vi "AlliGator Phasor ROI to Source Image ROI.vi"(8 "Error In":errorcluster, 10 "Phasor Plot ROI":T2, 11 "AlliGator IV DVR in":refnum<data-value>) -> (0 "Error Out":errorcluster, 1 "Message":string, 2 "Source Image ROI":T1 {"Contours"."Type" items=["No Selection", "Point", "Line", "Rectangle", "Oval", "Polygon", "Freehand Region", "Annulus", "Unused2", "Unused3", "Broken Line", "Freehand Line", "Rotated Rectangle"]}, 3 "AlliGator IV DVR out":refnum<data-value>, 4 "CPU (s)":dbl)   [LabVIEW 2021, in "AlliGator Phasor Plot.lvlib"]
doc: "Buils a Source Image ROI comprising all pixels whose phasors are included in the Phasor Plot ROI."
uses:
  AlliGator Phasor Plot.lvlib
  Internal Variables/AlliGator Internal Variables v2.ctl
  <vilib>/vision/Image Controls.llb/IMAQ Image.ctl
  Internal Variables/AlliGator Gate Image Set.ctl
  Files/AlliGator FLI Dataset Type.ctl
  Files/AlliGator Data Series Type.ctl
  Dual-Channel Datasets/AlliGator Dataset Channel.ctl
  Settings/AlliGator Gate Arithmetic.ctl
  Source Image/AlliGator Displayed Image.ctl
  Image/Named ROI Description.ctl
  Phasor Graph/AlliGator Decay Metadata v3.ctl
  Decay Analysis/Decay Preprocessing/AlliGator Decay Background Subtraction Info.ctl
  Decay Analysis/Decay Preprocessing/AlliGator Baseline Subtraction Method.ctl
  Graphs/XY Graph/XY Graph Plot Shift Parameters.ctl
  Graphs/XY Graph/XY Graph Plot Shift Method.ctl
  Decay Analysis/Decay Preprocessing/AlliGator Decay Extrapolation Parameters.ctl
  Phasor/Calibration Phasor (m, phi).ctl
  Phasor/Phasor Reference Series.ctl
  Phasor/Phasor Calibration Map v2.ctl
  Phasor/Phasor (g, s).ctl
  Phasor Graph/AlliGator Raw Phasor Plot Data v4.ctl
  Phasor/Phasor Standard Deviation Options.ctl
  AlliGator Phasor Multi-Harmonic Data.ctl
  Phasor/Phasor Harmonic Data.ctl
  Decay Fit Parameter Map/AlliGator Decay Fit Options & Parameters v2.ctl
  Fits/IRF(X)PSED/Decay Fit Options v2.ctl
  Fits/Decay Convolution/Decay Model.ctl
  Fits/Residual Type.ctl
  Fits/IRF(X)PSED/Fit Weights Type.ctl
  Fits/Non-linear Fitting Method v2.ctl
  Fits/Fit Calculation Method.ctl
  Fits/Non-linear Fitting Algorithm.ctl
  Decay Analysis/Decay Fit/AlliGator Decay Fit Parameter Constraints 2.ctl
  Fits/IRF(X)PSED/Decay Fit Parameters In List.ctl
  Fits/IRF(X)PSED/MLE Baseline Offset Type.ctl
  Decay Analysis/Decay Preprocessing/AlliGator Decay Preprocessing Parameters.ctl
  Fits/IRF(X)PSED/Decay Fit Parameters & Derived Quantities List v2.ctl
  Decay Fit Parameter Map/AlliGator Parameter Maps Data.ctl
  Globals, Variables, Constants/AlliGator Variables List.ctl
  Phasor Ratio/AlliGator Phasor Plot Reference Points.ctl
  9cfa6bdc-d1e0-4e6c-94b8-050a3d16fc11.vi
  <vilib>/vision/NI_Vision_Development_Module.lvlib
  Globals, Variables, Constants/AlliGator Globals, Variables & Constants.lvlib
  Phasor Ratio/AlliGator Phasor Ratio.lvlib
  Time/Time.lvlib
  Utilities/Utilities.lvlib
  Image/Image.lvlib
  Phasor/Phasor.lvlib
  Decay Analysis/Decay Preprocessing/AlliGator Decay Preprocessing.lvlib
  Graphs/XY Graph/XY Graph Add-Ons.lvlib
  Phasor Graph/AlliGator Phasor Graph.lvlib
  Files/AlliGator Files.lvlib
  Source Image/AlliGator Source Image.lvlib
  Internal Variables/AlliGator Internal Variables.lvlib
  Fits/Fits.lvlib
  Decay Analysis/Decay Fit/AlliGator Decay Fit.lvlib
  Decay Fit Parameter Map/AlliGator Decay Fit Parameter Map.lvlib
  Settings/AlliGator Settings.lvlib
  Dual-Channel Datasets/AlliGator Dual-Channel Datasets.lvlib
panel:
  # "see the AlliGator License on the block diagram (Ctrl+E or Window:Show Block Diagram)"
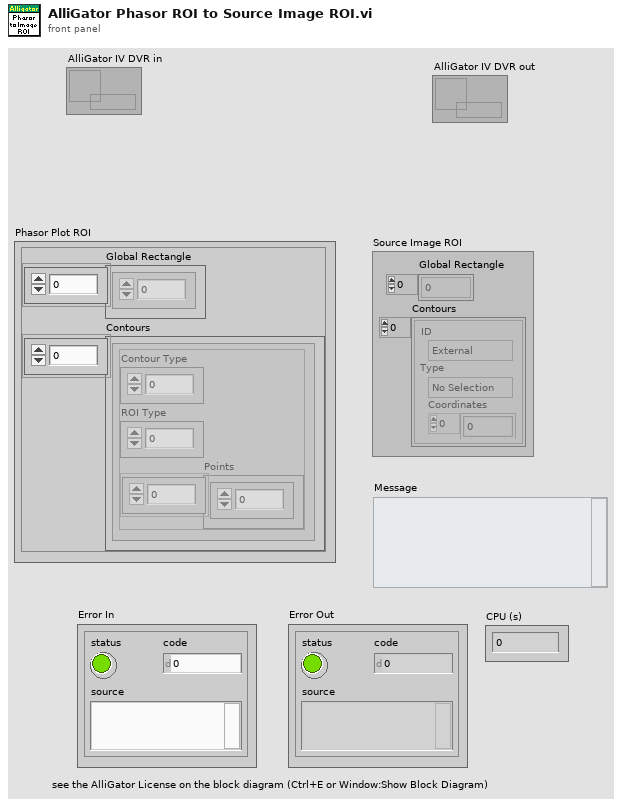
[diagram p1: front panel]
types:
  T1 = typedef "ROI Descriptor" = cluster{"Global Rectangle":i32[], "Contours":cluster{"ID":enum32{"External", "Internal"}, "Type":u32, "Coordinates":i32[]}[]}
  T2 = cluster{"Global Rectangle":i32[], "Contours":cluster{"Contour Type":u32, "ROI Type":u32, "Points":i32[]}[]}
  T3 = typedef "AlliGator Phasor Ratio.lvlib/AlliGator Phasor Plot Reference Points.ctl" = cluster{"O_h":dbl, "O_v":dbl, "1_h":dbl, "1_v":dbl}
  T4 = typedef "AlliGator Globals, Variables & Constants.lvlib/AlliGator Variables List.ctl" = enum16{"---- GUI ----", "GUI:Initialization Status", "GUI:State Indicators Refnum", "GUI:Original AlliGator Menu Items", "GUI:Current Action Loop State", "GUI:Script in progress", "GUI:Playback", "GUI:Loop Playback", "GUI:Search ROI Used", "GUI:Search ROI", "Decay Graph Max Legend Size", "Intensity Graph Max Legend Size", "Decay Statistics Graph Max Legend Size", "Phasor Graph Max Legend Size", "Phasor Ratio Graph Max Legend Size", "Lifetime Graph Max Legend Size", "---- Files ----", "Files:Export Dataset Frames as Individual Files", "Files:Show Batch Export Help Balloons", "Files:Frames in Dataset", "Files:ptu File Frame Start Indices", "Files:Current Frame in Dataset", "Files:Current Frame Timestamp", "Files:Dataset Loaded", "Files:Dataset Metadata", "Files:Dataset Channel", "Files:Dataset Data Description", "Files:Background Dataset Metadata", "Files:Background Dataset Channel", "Files:Background Dataset Data Description", "Files:Background File Subtraction", "Files:Background File Path", "Files:Background File Pile-up Correction", "Files:Background File Pixel Well Capacity", "Files:Background File Scaling Factor", "Files:Current Dataset Load Settings", "Files:Dataset Path", "Files:ICCD-specific Information", "Files:Macrotime Gate Separation", "------ Python Plugins ------", "Python Plugins:Information", "Python Plugins:Python Session", "Python Plugins:Valid Python Session?", "---- Source Image ----", "Source Image:ROIs", "Source Image:Current ROI", "Source Image:ROI Event Refnum", "X_Source Image Display Range", "X_Source Image Palette Information", "X_Type of Displayed Image", "X_Time Gate Slider", "Source Image:Palette List", "Source Image:Scale", "Source Image:ROI Overlay Color", "Source Image:Overlay to Erase", "Source Image:Is Displayed Image Accumulated", "Source Image:White Light Image Modified", "Source Image:Mask Image Modified", "---- Image Profile Window ----", "Image Profile:Window Event Refnum", "Image Profile:IntensityType", "Image Profile:Intensity Average Type", "Image Profile:Intensity-weighted SDV", "Image Profile:Box Profile Type", "Image Profile:Window Open", "Image Profile:Plotted Fit Parameter", "------ Phasor Graph -------", "Phasor Graph:Show Line", "---- Phasor Plot ---", "Phasor Plot:Parameters Changed", "Phasor Plot:FLI Dataset Modified since last Calculation", "Phasor Harmonics Data", "Selected Phasor Harmonics", "Phasor Harmonic Manager Event Refnum", "Phasor Plot:ROIs", "Phasor Plot:Current ROI", "Phasor Plot:ROI Event Refnum", "Phasor Plot:Image Reference Points", "Phasor Plot:Computed", "Phasor Plot:Palette Information", "Phasor Plot:Palette List", "Phasor Plot:Phasor Ratio Palette Information", "Phasor Plot:Phasor Ratio Palette List", "Phasor Plot:Image Scale", "Phasor Plot:Image Overlay to Erase", "Phasor Plot:Image Elements to Update", "Phasor Plot:Current Calculation Parameters", "Phasor Plot:Current Calibration Options", "Phasor Plot:Reset Cumulated Phasor Plot", "Phasor Plot:Reference 1", "Phasor Plot:Lifetime Reference 1", "Phasor Plot:Reference 1 Frequency", "Phasor Plot:Reference 2", "Phasor Plot:Lifetime Reference 2", "Phasor Plot:Reference 2 Frequency", "---- Decay Analysis ----", "Number of Selected Decays to Fit", "LS Fit Results", "LAR Fit Results", "BS Fit Results", "Last Decay Max - Min", "Best Fit Parameters", "Best Fit Parameter Names", "Actual Size X", "Actual Size Y", "Binning X", "Binning Y", "Actual # Gates", "Dataset Number", "Gates to...", "Gates Skipped", "Gates to keep", "Gate Step", "Gate Separation", "Reversed Gates", "Pile-up Correction", "Pixel Well Capacity", "Background Subtracted", "Background Subtraction Method", "Background Definition Range", "Background File (deprecated)", "Number of Dataset Accumulated", "Array of Accumulated Dataset Paths", "Do Averaged Datasets", "Destination File Path", "Process Plot Target", "Use 1/D as Phasor Frequency", "---- Decay Fit Parameter Map -----", "Decay Fit Parameter Map:Palette Information", "Decay Fit Parameter Map:Palette List", "---- Parameter Map ----", "Parameter Map:Palette Information", "Parameter Map:Palette List", "------- Local Decay Window ---------", "Local Decay Graph Window:Event Refnum", "Local Decay Graph Window:Use normalized IRF for convolution", "----- Miscellaneous ----", "Misc:Skippable Dialog Windows Status"}
  T5 = typedef "AlliGator Internal Variables.lvlib/AlliGator Internal Variables v2.ctl" = cluster{"Displayed Image":T6, "White Light Image":T6, "Mask Image":T6, "ROI Mask Image":T6, "Current Dataset Images 1":T7, "Background Dataset Images 1":T7, "Current Dataset Images 2":T7, "Background Dataset Images 2":T7, "Current Dataset Arithmetic Images":T7, "Accumulated Dataset Images 1":T7, "Accumulated Dataset Images 2":T7, "Accumulated Dataset Arithmetic Images":T7, "Phasor Plot Image":T6, "Decay Fit Parameter Map Image":T6, "Parameter Map Image":T6, "Single Data Point Path":path, "White Light Image Path":path, "Mask Image Path":path, "Time-Series Folder":path, "[Time-Series Paths]":path[], "Current Dataset":i32, "Single Dataset Type":T8, "Current Folder":string, "AlliGator Data Series Type":T9, "# Datasets":i32, "Dual-Channel Dataset":bool, "Selected Channel Name":string, "Dataset Channel":T10, "Channel Arithmetic":T11, "Dual-Channel Background Dataset":bool, "Background Channel":T10, "Dual-Channel Accumulated Dataset":bool, "Start Time":dbl, "[Time-Series Timestamps]":dbl[], "[Intensity Corrections]":dbl[], "Time Series Script":bool, "Type of Displayed Image":T12, "Gate Image Slide":u16, "# Gates":i32, "ROIs":T13[], "ROI Decay":cluster{"t Array":dbl[], "I Array":dbl[]}, "Valid Decay":bool, "Decay  Metadata":T14, "Reference Decay Plot Name":string, "Reference Decay":cluster{"t Array":dbl[], "I Array":dbl[]}, "Decay Shift Plot":cluster{"Time Stamps":dbl[], "Decay Shifts":dbl[]}, "[Decays Max Values]":sgl[], "[Decays Min Values]":sgl[], "Calibration Phasor":T20, "Calibration Phasor Series":T21, "Phasor Calibration Map":T22, "Calibration Map MD5 Digest":string, "Last Raw Phasor":T23, "Last Calibrated Phasor":T23, "Last Calibrated Phasor SDV":T23, "Phasor Graph:Phasor Plot":cluster{"g Array":dbl[], "s Array":dbl[]}, "Phasor Graph:Phasor SDV Plot":cluster{"g Array":dbl[], "s Array":dbl[]}, "[Phasor Graph:Raw Phasor Plots]":T24[], "Phasor Plot locked to Ref 1":i32, "[Phasor Plot(s) locked to Ref 1]":i32[], "[Phasor Plot(s) locked to Ref 2]":i32[], "[Pixel Phasors]":T23[], "[[Sum Image]]":dbl[][], "[[CSG Phasors]]":csg[][], "[[Valid Pixel?]]":bool[][], "I/m/phi Dataset":cluster{"I/m/phi Dataset?":bool, "Base Frequency":dbl[unit], "Harmonic Orders":u8[]}, "Multi Phasor Plot Data":T26, "Decay Fit Options & Parameters":T28, "Fit Options: Decay Preprocessing Parameters":T39, "Fit Options: Reference Decay":cluster{"t Array":dbl[], "I Array":dbl[]}, "Is Full Image Parameters Map":bool, "Is Single-Pixels Parameters Map":bool, "NLSF Parameters Map X Resolution":i32, "NLSF Parameters Map Y Resolution":i32, "[Single Decay Fit Parameters]":dbl[], "Fit Model":T30, "[[Multiple Decays Fit Parameters]]":dbl[][], "[[Multiple Decays Fit Parameter SDVs]]":dbl[][], "[[IRFs]]":dbl[][], "IRF Array Time Axis":dbl[], "Decay Array Time Axis":dbl[], "[Decay Fit Parameter Names]":T40[], "[[Phasor Ratios]]":dbl[][], "[[Average Lifetimes]]":dbl[][], "Amplitude Weighted Average Lifetime":bool, "[Decay Sum]":dbl[], "[Map Set Names]":string[], "[Parameter Maps]":T41[], "[[User-defined Quantities]]":dbl[][], "User-defined Quantity":string}
  T6 = typedef "IMAQ Image.ctl" = refnum<image>
  T7 = typedef "AlliGator Internal Variables.lvlib/AlliGator Gate Image Set.ctl" = cluster{"SGL Image Max":T6, "SGL Image Sum":T6, "SGL Gate Images":T6[], "SGL Image Min":T6}
  T8 = typedef "AlliGator Files.lvlib/AlliGator FLI Dataset Type.ctl" = enum16{"HDF5 FLI Dataset", "Gate Image Folder", ".sdt FLI Dataset (Becker & Hickl)", ".ptu FLI Dataset (PicoQuant)", "SS1 FLI Dataset", "SS2 FLI Dataset", "I/m/phi Dataset", ".bin FLI Dataset (PicoQuant Binned)", ".bin FLI Dataset (Piccolo Binned)"}
  T9 = typedef "AlliGator Files.lvlib/AlliGator Data Series Type.ctl" = enum16{"Not a Supported Series", "Gate Images Folder Series", "SwissSPAD 2 Dataset Series", "B&H FLI Dataset Series", "PicoQuant PTU FLI Dataset Series", "PicoQuant BIN FLI Dataset Series", "Piccolo hist BIN FLI Dataset Series", "HDF5 FLI Dataset Series"}
  T10 = typedef "AlliGator Dual-Channel Datasets.lvlib/AlliGator Dataset Channel.ctl" = enum16{"G2", "INT"}
  T11 = typedef "AlliGator Settings.lvlib/AlliGator Gate Arithmetic.ctl" = enum16{"None", "INT-G2", "G2/INT*<INT>", "(1 - G2/INT)*<INT>"}
  T12 = typedef "AlliGator Source Image.lvlib/AlliGator Displayed Image.ctl" = enum16{"Single Gate", "Sum of All Gates", "Max of All Gates", "Min of All Gates", "-", "White Ligth Image", "Mask Image"}
  T13 = typedef "Image.lvlib/Named ROI Description.ctl" = cluster{"ROI Descriptor":T1, "ROI Name":string, "Overlay Color":u32}
  T14 = typedef "AlliGator Phasor Graph.lvlib/AlliGator Decay Metadata v3.ctl" = cluster{"ROI Descriptor":T1, "ROI Center":cluster{"X":i32, "Y":i32}, "Decay Background Subtraction Info":T15, "Decay Reverted":bool, "Decay Smoothened":bool, "Decay Straightened":bool, "Fitted Tau (Decay Straightening)":dbl, "Decay Shift Parameters":T17, "Decay Shifted":bool, "Decay Extrapolated":bool, "Decay Extrapolation Parameters":T19, "Decay Normalized":bool, "Fold Decay":bool, "# Folds":u32}
  T15 = typedef "AlliGator Decay Preprocessing.lvlib/AlliGator Decay Background Subtraction Info.ctl" = cluster{"Laser Period":dbl[unit], "Gate Duration":dbl[unit], "Baseline Subtraction Method":T16, "Background Definition Range":cluster{"Min Gate":dbl[unit], "Max Gate":dbl[unit]}, "Total Intensity w/o Bkgd Subtraction":dbl, "Bkgd-subtracted Intensity (exp)":dbl, "# Data Points":i32, "Background/Gate":dbl, "Fitted Lifetime":dbl[unit], "Bkgd-subtracted Intensity (theo)":dbl}
  T16 = typedef "AlliGator Decay Preprocessing.lvlib/AlliGator Baseline Subtraction Method.ctl" = enum16{"Mean", "Min", "Square Gated Single-Exponential", "File", "Constant"}
  T17 = typedef "XY Graph Add-Ons.lvlib/XY Graph Plot Shift Parameters.ctl" = cluster{"Type":T18, "Shift":dbl[unit], "Threshold":dbl, "Rotate":bool}
  T18 = typedef "XY Graph Add-Ons.lvlib/XY Graph Plot Shift Method.ctl" = enum16{"Default", "CFD", "Threshold", "Cross-Correlation"}
  T19 = typedef "AlliGator Decay Preprocessing.lvlib/AlliGator Decay Extrapolation Parameters.ctl" = cluster{"Additional Points":u32, "Head Fraction":dbl, "Fitted Tau":dbl, "Use Periodicity":bool, "Use Cursors":bool, "Tail Fraction":dbl}
  T20 = typedef "Phasor.lvlib/Calibration Phasor (m, phi).ctl" = cluster{"m":dbl, "phi":dbl, "Phasor Frequency":dbl[unit], "Reference Lifetime":dbl[unit]}
  T21 = typedef "Phasor.lvlib/Phasor Reference Series.ctl" = cluster{"m Array":dbl[], "phi Array":dbl[], "Phasor Frequency":dbl[unit], "Calibration Lifetime":dbl[unit]}
  T22 = typedef "Phasor.lvlib/Phasor Calibration Map v2.ctl" = cluster{"Phasor Frequency":dbl[unit], "Calibration Lifetime":dbl[unit], "ROI Centers":cluster{"X":i32, "Y":i32}[], "ROI Descriptors":T1[], "Map Resolution X":i32, "Map Resolution Y":i32, "z Array":cdb[]}
  T23 = typedef "Phasor.lvlib/Phasor (g, s).ctl" = cluster{"g":dbl, "s":dbl}
  T24 = typedef "AlliGator Phasor Graph.lvlib/AlliGator Raw Phasor Plot Data v4.ctl" = cluster{"Phasor Plot Name":string, "Raw Phasor Plot":T23[], "Phasor Frequency":dbl[unit], "[Decay Metadata]":T14[], "Raw Phasor Plot SDV":T23[], "Phasor SDV Options":T25, "[Calibration Phasor]":T20[]}
  T25 = typedef "Phasor.lvlib/Phasor Standard Deviation Options.ctl" = cluster{"Compute Estimated SDV":bool, "# Replicas":u32, "Use Estimated Average Phasor":bool}
  T26 = typedef "AlliGator Phasor Plot.lvlib/AlliGator Phasor Multi-Harmonic Data.ctl" = cluster{"Base Frequency":dbl[unit], "# Harmonics":u8, "Harmonic Orders":u8[], "Phasor Plot Settings Checksum":u64, "Phasor Harmonic Data Array":T27[]}
  T27 = typedef "Phasor.lvlib/Phasor Harmonic Data.ctl" = cluster{"Phasor Harmonic Name":string, "Phasor Plot Settings Checksum":u64, "Phasor Frequency":dbl[unit], "Base Frequency":dbl[unit], "Harmonic Order":u8, "Phasor Plot Parameters":string, "Phasor Array [[CSG]]":csg[][], "Dataset File Path":path}
  T28 = typedef "AlliGator Decay Fit Parameter Map.lvlib/AlliGator Decay Fit Options & Parameters v2.ctl" = cluster{"SYNC Period":dbl[unit], "Fit Options":T29, "Fit Parameter Constraints":T36[], "MLE Baseline Offset":dbl, "MLE Baseline Offset Type":T38}
  T29 = typedef "Fits.lvlib/Decay Fit Options v2.ctl" = cluster{"Show Fit Residuals":bool, "Fit Model":T30, "Residual Type":T31, "Max Decay Percentile":dbl, "Min Decay Percentile":dbl, "Show Full Decay":bool, "Weights":T32, "Fitting Method":T33, "Compute Parameter Uncertainties":bool, "Periodic Boundaries":bool, "Model Calculation":T34, "Period":dbl[unit], "Termination Criteria":cluster{"Max Iterations":i32, "Max Function Calls":i32, "Max Time":dbl[unit], "Function Tolerance":dbl, "Parameter Tolerance":dbl, "Gradient Tolerance":dbl, "Min Lambda":dbl, "Max Lambda":dbl, "Initial Tick Count":u32}, "Offset Resolution":dbl[unit], "Use Local IRF":bool, "Fitting Algorithm":T35}
  T30 = typedef "Fits.lvlib/Decay Model.ctl" = enum16{"1-Exponential", "2-Exponentials"}
  T31 = typedef "Fits.lvlib/Residual Type.ctl" = enum16{"Standard", "Normalized", "Reduced"}
  T32 = typedef "Fits.lvlib/Fit Weights Type.ctl" = enum16{"Unweighted", "1/Variance", "Best of All"}
  T33 = typedef "Fits.lvlib/Non-linear Fitting Method v2.ctl" = enum16{"Least Square", "Least Absolute Residual", "Bisquare", "MLE", "-", "Best of All"}
  T34 = typedef "Fits.lvlib/Fit Calculation Method.ctl" = enum16{"Simulation", "Convolution", "Integration"}
  T35 = typedef "Fits.lvlib/Non-linear Fitting Algorithm.ctl" = enum16{"Levenberg-Marquardt", "Trust-Region Dogleg"}
  T36 = typedef "AlliGator Decay Fit.lvlib/AlliGator Decay Fit Parameter Constraints 2.ctl" = cluster{"Fit Parameter":T37, "Min Value":dbl, "Max Value":dbl, "Global":bool, "Used":bool}
  T37 = typedef "Fits.lvlib/Decay Fit Parameters In List.ctl" = enum16{"Offset", "Baseline", "A_1", "tau_1", "A_2", "tau_2"}
  T38 = typedef "Fits.lvlib/MLE Baseline Offset Type.ctl" = enum32{"Absolute", "Percentage"}
  T39 = typedef "AlliGator Decay Preprocessing.lvlib/AlliGator Decay Preprocessing Parameters.ctl" = cluster{"Background Subtraction":bool, "Straighten Decay":bool, "Reverse Gates":bool, "1-Normalized Decay":bool, "Smoothen Decay":bool, "Smoothing Parameter":dbl, "Shift Decay":bool, "Decay Shift Parameters":T17, "Extrapolate Decay":bool, "Additional Points":u32, "Head Fraction":dbl, "Pixel-Normalize Decay":bool, "Use Periodicity":bool, "Use Cursors":bool, "Tail Fraction":dbl, "Use Decay Pre-Processing":bool, "Fold Decay":bool, "# Folds":u32, "[0-1]-Normalized Decay":bool}
  T40 = typedef "Fits.lvlib/Decay Fit Parameters & Derived Quantities List v2.ctl" = enum16{"Offset", "Baseline", "A_1", "tau_1", "A_2", "tau_2", "<tau>_a", "f1_a", "f2_a", "<tau>_i", "f1_i", "f2_i", "-", "R^2", "Chi^2"}
  T41 = typedef "AlliGator Decay Fit Parameter Map.lvlib/AlliGator Parameter Maps Data.ctl" = cluster{"Map Set Name":string, "[Parameter Names]":string[], "[[Parameters]]":dbl[][], "[[Parameter SDVs]]":dbl[][], "Decay Array Time Axis":dbl[], "[[IRFs]]":dbl[][], "IRF Array Time Axis":dbl[]}
  T42 = typedef "Image Type" = u32
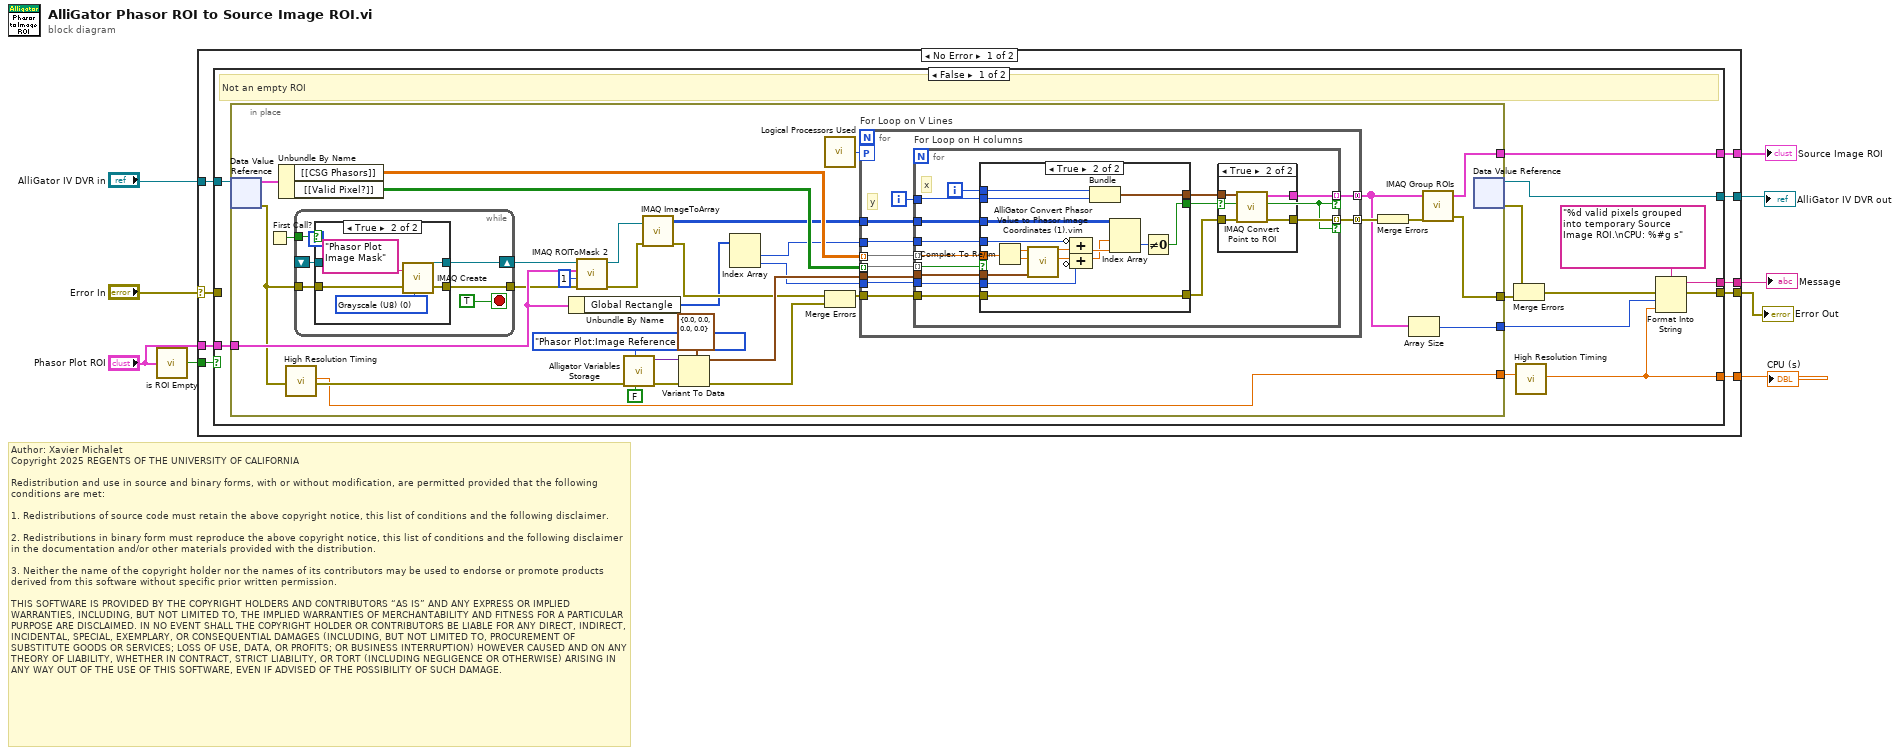
[diagram p0: block diagram]
diagram:
  # "Author: Xavier Michalet\nCopyright 2025 REGENTS OF THE UNIVERSITY OF CALIFORNIA\n\nRedistribution and use in source and binary forms, with or without modification, are permitted provided that the following conditions are met:\n\n1. Redistributions of source code must retain the above copyright notice, this list of conditions and the following disclaimer.\n\n2. Redistributions in binary form must reproduce the above copyright notice, this list of conditions and the following disclaimer in the documentation and/or other materials provided with the distribution.\n\n3. Neither the name of the copyright holder nor the names of its contributors may be used to endorse or promote products derived from this software without specific prior written permission.\n\nTHIS SOFTWARE IS PROVIDED BY THE COPYRIGHT HOLDERS AND CONTRIBUTORS “AS IS” AND ANY EXPRESS OR IMPLIED WARRANTIES, INCLUDING, BUT NOT LIMITED TO, THE IMPLIED WARRANTIES OF MERCHANTABILITY AND FITNESS FOR A PARTICULAR PURPOSE ARE DISCLAIMED. IN NO EVENT SHALL THE COPYRIGHT HOLDER OR CONTRIBUTORS BE LIABLE FOR ANY DIRECT, INDIRECT, INCIDENTAL, SPECIAL, EXEMPLARY, OR CONSEQUENTIAL DAMAGES (INCLUDING, BUT NOT LIMITED TO, PROCUREMENT OF SUBSTITUTE GOODS OR SERVICES; LOSS OF USE, DATA, OR PROFITS; OR BUSINESS INTERRUPTION) HOWEVER CAUSED AND ON ANY THEORY OF LIABILITY, WHETHER IN CONTRACT, STRICT LIABILITY, OR TORT (INCLUDING NEGLIGENCE OR OTHERWISE) ARISING IN ANY WAY OUT OF THE USE OF THIS SOFTWARE, EVEN IF ADVISED OF THE POSSIBILITY OF SUCH DAMAGE."
  n1 = call "is ROI Empty.vi"("Current ROI Descriptor"="Phasor Plot ROI") -> ("Empty ROI?"=w6:bool)  [unwired: 8 in]
  n2 = case shown="No Error" "Error In" {
    selector: "Error In" -> [w12 w127]
    tunnel: "AlliGator IV DVR in" -> [w18 w128]
    tunnel: [w17 w128] -> w8
    tunnel: [w16 w127] -> w7
    tunnel: w6 -> [w15 _]
    tunnel: [w14 _] -> w5
    tunnel: "Phasor Plot ROI" -> [w13 _]
    tunnel: [w11 _] -> w2
    tunnel: [w10 _] -> w1
    frame No Error {
      n3 = case shown="False" w15 {
        tunnel: w18 -> [w30 w126]
        tunnel: [w29 w126] -> w17
        tunnel: [w23 w125] -> w16
        tunnel: w13 -> [w26 _]
        tunnel: [w20 _] -> w14
        tunnel: w12 -> [_ w125]
        tunnel: [w24 _] -> w11
        tunnel: [w19 _] -> w10
        frame False {
          # "Not an empty ROI"
          n4 = in-place {
            in-place-border: [w35] -> w31
            in-place-border: [w38] -> w25
            in-place-border: w26 -> [w63]
            in-place-border: [w34] -> w24
            in-place-border: [w32] -> w22
            n5 = in-place-dvr #1(w30) -> (w64:T5, w40:errorcluster)
            n6 = First Call?() -> (First Call?: T/F=w59:bool)
            n7 = Unbundle By Name(w64) -> ("[[CSG Phasors]]"=w61:csg[][], "[[Valid Pixel?]]"=w62:bool[][])
            n8 = call "High Resolution Timing.vi"("Error In"=w40) -> ("elapsed (relative) seconds"=w38:dbl, "Error Out"=w41:errorcluster)  [unwired: 16 in, 1 out]
            n9 = while {
              tunnel: w59 -> [w117]
              tunnel: w40 -> [w116]
              shift-right: [w115] -> w42
              shift-left: _ -> [w113]
              tunnel: [w112] -> w44
              stop <- TRUE stop-if-true
              n10 = case shown="True" w117 {
                tunnel: w116 -> [w118 w123]
                tunnel: [w119 w122] -> w115
                tunnel: w113 -> [w119 _]
                tunnel: [w118 w121] -> w112
                frame False {
                }
                frame True {
                  w120 = T42 0 items=["Grayscale (U8)", "Grayscale (I16)", "Grayscale (SGL)", "Complex (CSG)", "RGB (U32)", "HSL (U32)", "RGB (U64)", "Grayscale (U16)"] ("Image Type")
                  n11 = call "IMAQ Create"("Image Name"="Phasor Plot Image Mask", "Image Type"=w120, "error in (no error)"=w123) -> ("New Image"=w122:T6, "error out"=w121:errorcluster)  [unwired: 2 in]
                }
              }
            }
            n12 = Unbundle By Name(w63) -> ("Global Rectangle"=w48:i32[])
            n13 = call "IMAQ ROIToMask 2"("error in (no error)"=w44, "Filling Value (255)"=1, "ROI Descriptor"=w63, "Image"=w42) -> ("error out"=w43:errorcluster, "Image Out"=w51:T6)  [unwired: 5 in, 1 out]
            n14 = call "Alligator Variables Storage.vi"("Get(F)/Set"=FALSE, "AlliGator Variable"=AlliGator_Variables_List."Phasor Plot:Image Reference Points" ("Alligator Variable"), "Error In"=w41) -> ("Error Out"=w54:errorcluster, "Data out"=w56:variant)  [unwired: 6 in, 1 out]
            n15 = call "IMAQ ImageToArray"("error in (no error)"=w43, "Image"=w51) -> ("error out"=w49:errorcluster, "Image Pixels (U8)"=w50:u8[][])  [unwired: 2 in, 3 out]
            n16 = Variant To Data(error in=w54, type=T3 {"O_h"=0.0, "O_v"=0.0, "1_h"=0.0, "1_v"=0.0} ("Phasor Plot Reference Points"), Variant=w56) -> (data=w53:T3, error out=w39:errorcluster)
            n17 = Index Array(array=w48) -> (element #1=w47:i32, element #2=w46:i32)  [unwired: 2 in]
            n18 = call "Logical Processors Used.vi"() -> ("# Logical Processor Used"=w45:i32)  [unwired: 6 in]
            n19 = Merge Errors(w49, w39) -> (w52:errorcluster)
            n20 = for "For Loop on V Lines" {
              tunnel: w61 -> [w74] mode=indexing
              tunnel: w53 -> [w72]
              tunnel: w47 -> [w71]
              tunnel: w46 -> [w70]
              tunnel: w52 -> [w69]
              tunnel: w62 -> [w68] mode=indexing
              workers-P: w45 -> [_]
              tunnel: w50 -> [w67]
              tunnel: [w66] -> w33 mode=concatenating
              tunnel: [w65] -> w37 mode=concatenating
              i -> [w73]
              # "y"
              n21 = for "For Loop on H columns" {
                tunnel: w74 -> [w88] mode=indexing
                tunnel: w73 -> [w84]
                tunnel: w72 -> [w87]
                tunnel: w71 -> [w86]
                tunnel: w70 -> [w85]
                tunnel: w69 -> [w82]
                tunnel: w68 -> [w81] mode=indexing
                tunnel: w67 -> [w80]
                tunnel: [w77] -> w66 mode=indexing if=w75
                tunnel: [w76] -> w65 mode=indexing if=w75
                i -> [w83]
                # "x"
                n22 = case shown="True" w81 {
                  tunnel: w88 -> [_ w108]
                  tunnel: w87 -> [_ w106]
                  tunnel: w86 -> [_ w102]
                  tunnel: w85 -> [_ w101]
                  tunnel: w84 -> [_ w97]
                  tunnel: w83 -> [_ w98]
                  tunnel: [_ w95] -> w79
                  tunnel: [w94 w100] -> w78
                  tunnel: w82 -> [w94 w100]
                  tunnel: [_ w99] -> w75
                  tunnel: w80 -> [_ w96]
                  frame False {
                  }
                  frame True {
                    n23 = Complex To Re/Im(x + iy=w108) -> (x=w109:sgl, y=w107:sgl)
                    n24 = call "AlliGator Convert Phasor Value to Phasor Image Coordinates (1).vim"("Phasor Plot Reference Points"=w106, "Phasor s"=w107, "Phasor g"=w109) -> ("Phasor Plot y"=w111:dbl, "Phasor Plot x"=w104:dbl)  [unwired: 7 in]
                    n25 = Compound Arithmetic op=ADD(invert w102, w104) -> (w105:dbl)
                    n26 = Compound Arithmetic op=ADD(w111, invert w101) -> (w103:dbl)
                    n27 = Bundle(w98, w97) -> (w95:cluster{i32, i32})  [unwired: 1 in]
                    n28 = Index Array(array=w96, index (row)=w103, index (col)=w105) -> (element=w110:u8)
                    n29 = Not Equal To 0?(x=w110) -> (x != 0?=w99:bool)
                  }
                }
                n30 = case shown="True" w75 {
                  tunnel: w79 -> [_ w93]
                  tunnel: w78 -> [w89 w92]
                  tunnel: [_ w91] -> w77
                  tunnel: [w89 w90] -> w76
                  frame False {
                  }
                  frame True {
                    n31 = call "IMAQ Convert Point to ROI"("error in (no error)"=w92, "Point"=w93) -> ("error out"=w90:errorcluster, "ROI Descriptor"=w91:T1)  [unwired: 7 in]
                  }
                }
              }
            }
            n32 = Merge Errors(w37) -> (w36:errorcluster)
            n33 = Array Size(array=w33) -> (size(s)=w32:i32)
            n34 = call "IMAQ Group ROIs"("error in (no error)"=w36, "ROI Descriptors"=w33) -> ("error out"=w35:errorcluster, "ROI Descriptor out"=w34:T1)  [unwired: 2 in]
            n35 = in-place-dvr #1() -> (w29:refnum<data-value>, w27:errorcluster)  [unwired: 1 in]
          }
          n36 = Merge Errors(w27, w31) -> (w28:errorcluster)
          n37 = call "High Resolution Timing.vi"("relative seconds (NaN)"=w25) -> ("elapsed (relative) seconds"=w20:dbl)  [unwired: 16 in, 2 out]
          n38 = Format Into String(format string="%d valid pixels grouped into temporary Source Image ROI.\nCPU: %#g s", error in=w28, w22, w20) -> (resulting string=w19:string, error out=w23:errorcluster)  [unwired: 1 in]
        }
        frame True {
        }
      }
    }
    frame Error {
    }
  }
  "Error Out" <- w7
  "CPU (s)" <- w5
  "AlliGator IV DVR out" <- w8
  "Source Image ROI" <- w2
  "Message" <- w1
